vi "GT Get Capture Repeat Pos.vi"(6 "count":i16, 7 "startNum":i16, 8 "error in (no error)":errorcluster caption="错误输入（无错误）", 9 "pValue":i16[](array[numeric]), 10 "encoder":i16, 11 "cardNum":i16) -> (0 "error out":errorcluster caption="错误输出", 1 "pValue out":i16[](array[numeric]), 3 "function return":i16)   [LabVIEW 2014, in "gts.lvlib"]
doc: "GT_API GT_GetCaptureRepeatPos(short cardNum,short encoder,long *pValue,short startNum,short count);"
uses:
  gts.lvlib
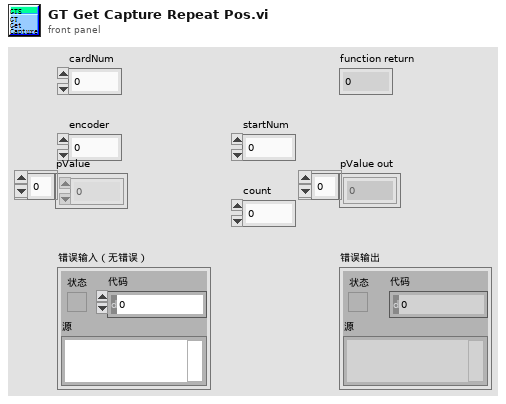
[diagram p1: front panel]
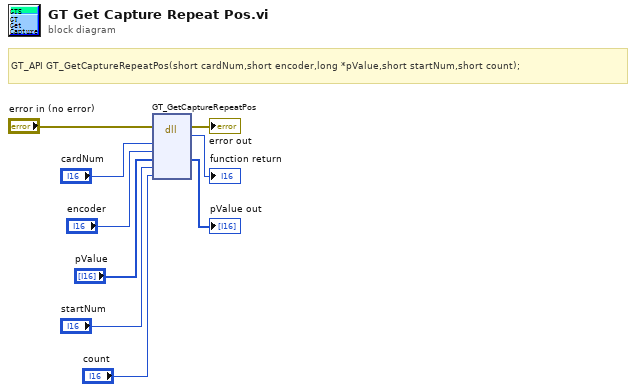
[diagram p0: block diagram]
diagram:
  # "GT_API GT_GetCaptureRepeatPos(short cardNum,short encoder,long *pValue,short startNum,short count);"
  n1 = dll-call lib="PTH2habs D固高科技资料GTS控制卡GTS卡18年上半年资料dllVC32bit\nmulti_cardgts.*" fn="GT_GetCaptureRepeatPos"(error in="error in (no error)", "cardNum"="cardNum", "encoder"="encoder", "pValue"="pValue", "startNum"="startNum", "count"="count") -> (error out=→"error out":errorcluster, "返回类型"=→"function return":i16, "pValue"=→"pValue out":i32[])  [unwired: 6 in, 1 out]
